vi "Read Ch Select.vi"(8 "error in (no error)":errorcluster, 11 "Lakeshore 325 in":refnum<class "Lakeshore 325.lvclass">) -> (0 "error out":errorcluster, 2 "Ch Select":i32[](array[numeric]), 3 "Lakeshore 325 out":refnum<class "Lakeshore 325.lvclass">)   [LabVIEW 2022 SP3, in "Lakeshore 325.lvclass"]
uses:
  Lakeshore 325.lvclass
  Lakeshore 325.lvclass/Lakeshore 325.ctl
  Temp Control.lvclass
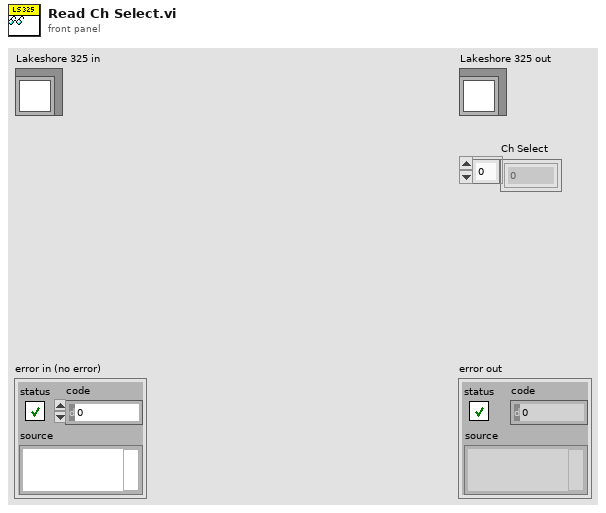
[diagram p1: front panel]
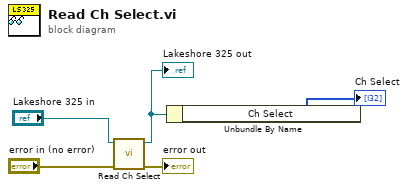
[diagram p0: block diagram]
diagram:
  n1 = call-parent "Read Ch Select.vi"("error in (no error)"="error in (no error)", "Temp Control in"="Lakeshore 325 in") -> ("error out"=→"error out":errorcluster, "Temp Control out"=w2:refnum<class "Lakeshore 325.lvclass">)  [unwired: 7 in, 1 out]
  "Lakeshore 325 out" <- w2
  n2 = Unbundle By Name(w2) -> ("Ch Select"=→"Ch Select":i32[])
